vi "PDF_Interface_PDF Protokoll Linearisierung.vi"(2 "ResultPictures":T1, 3 "PDF Optionen":T2, 4 "Deckblatt_Name":string, 5 "start":bool, 6 "SpanComponentInfos-Cluster":T7, 7 "Save PDF File Path":path, 8 "error in (no error)":errorcluster caption="Fehler (Eingang, kein Fehler)", 9 "Context (Eingang)":refnum<class "Context.lvclass">, 10 "XY-Graph LIN":refnum<vi>, 11 "Polynom-Ordnung":T8) -> (0 "error out":errorcluster caption="Fehler (Ausgang)", 1 "Context (Ausgang)":refnum<class "Context.lvclass">)   [LabVIEW 2020, in "Linearisierung v2.lvlib" / "Protokoll.lvlib"]
uses:
  Protokoll.lvlib
  AktivArray.ctl
  AktivButton.ctl
  LIN Ausgabetabelle.ctl
  Polynomkoeffizientenanzeige.ctl
  Auswahl Polynom Ordnung.ctl
  <vilib>/Simplicity AI/SAI_PDF_API/Classes/Context/Context.lvclass
  SpanEinstellungen/SpanComponentInfos-Cluster.ctl
  SpanEinstellungen/ComponentInfos.ctl
  Visualisierungs Elemente/String - Ausgabefeld.ctl
  Visualisierungs Elemente/String - Eingabefeld.ctl
  SpanEinstellungen/PDF Optionen.ctl
  PDF_Interface/PDF Interface Helper/PDFResultPictures.ctl
  Sprachverwaltung/FGV Aktion Tabelle zerlegen.ctl
  Aktion Lin Daten aufarbeiten.ctl
  Seiten/FT-IR/FGV FT-IR Gasliste Aktionen.ctl
  Seiten/System Einstellungen V2/Aktion FGV SystemEinstellungenV2.ctl
  Gasteiler/Aktionen FGV Gasteiler Daten.ctl
  Seiten/System Einstellungen V2/Aktioen FGV System Konstanten.ctl
  Seiten/FT-IR/FGV FT-IR Aktionen.ctl
  PDF_Interface/PDF Protokoll Standard Kopf Optionen.ctl
  <vilib>/Simplicity AI/SAI_PDF_API/Classes/Context/Controls/SAI_PDF_PDF Details.ctl
  PDF_Interface/PDF Interface Helper/PDFGraph.ctl
  <vilib>/Simplicity AI/SAI_PDF_API/Classes/Context/Controls/SAI_PDF_Text Align.ctl
  PDF_Interface/PDF Interface Helper/PDFCommentPosition.ctl
  PDF_Interface/PDF Interface Helper/PDFPageBreak.ctl
  PDF_Interface/PDF Interface Helper/PDFContentType.ctl
  PDF_Interface/PDF Interface Helper/PDFTableContentType.ctl
  PDF_Interface/PDF Interface Helper/PDFResults.ctl
  PDF_Interface/PDF Interface Helper/PDFTablePictures.ctl
  PDF_Interface/PDF Interface Helper/PDFBemerkung.ctl
  <vilib>/Simplicity AI/SAI_PDF_API/Classes/Context/Controls/SAI_PDF_Font.ctl
  <vilib>/Simplicity AI/SAI_PDF_API/Classes/Context/Controls/SAI_PDF_Font Encoding.ctl
  PDF_Interface/PDF Interface Helper/PDFTtilePageContentType.ctl
  Gasteiler/HovaCAL_Interface/Kommunikation/Aktion FGV HovaCAL Interface Autolin.ctl
  GasteilerType.ctl
  Linearisierung v2.lvlib
  Allgemein/allgemeine Sub-VIs.lvlib
  Seiten/FT-IR/FT-IR.lvlib
  Seiten/System Einstellungen V2/System Einstellungen V2.lvlib
  Sprachverwaltung/Sprachverwaltung.lvlib
  PDF_Interface/PDF Interface.lvlib
  PDF_Interface/PDF Interface Helper/PDF Interface Helper.lvlib
  Gasteiler/Gasteiler.lvlib
  Gasteiler/HovaCAL_Interface/Kommunikation/Kommunikation.lvlib
  SpanEinstellungen/SpanEinstellungen.lvlib
panel:
  out "Gasflaschengenauigkeit":string caption="Genauigkeit:"
  out "Gasflaschennummer":string caption="Gasflasche:"
  out "Spanfaktor":string caption="Spanfaktor:"
  out "geforderte Genauigkeit":string caption="geforderte Genauigkeit:"
  out "Polynomkoeffizienten":T9 caption="Polynomkoeffizient:" {"O. 4" format="%#.10f"; "O. 3" format="%#.10f"; "O. 2" format="%#.10f"; "O.1" format="%#.10f"; "Offset" format="%#.10f"}
  out "Polynom-Ordnung":string caption="Polynom-Ordnung:"
  out "Ordnung festgelegt":string caption="Ordnung festgelegt:"
  out "erreichter max. Fehler (ppm)":string caption="erreichter max. Fehler (ppm):"
  out "erreichter max. Fehler (%)":string caption="erreichter max. Fehler (%):"
  out "geford. max. Fehler":string caption="geford. max. Fehler (% v. Sollw.):"
  out "LIN Ausgabetabelle":T10
  out "Aktiv":T11
  out "XY-Graph LIN":cluster{dbl[], dbl[]}[](graph) caption="XY-Graph"
  out "Datum:":string
  out "Konzentration:":string
  out "Komponente:":string
  out "Bearbeiter:":string
  out "Gasteiler:":string
  out "Messgerät:":string
  # "Linearity Check"
  # "Konstante"
  # "1.Ordnung"
  # "2.Ordnung"
  # "3.Ordnung"
  # "4.Ordnung"
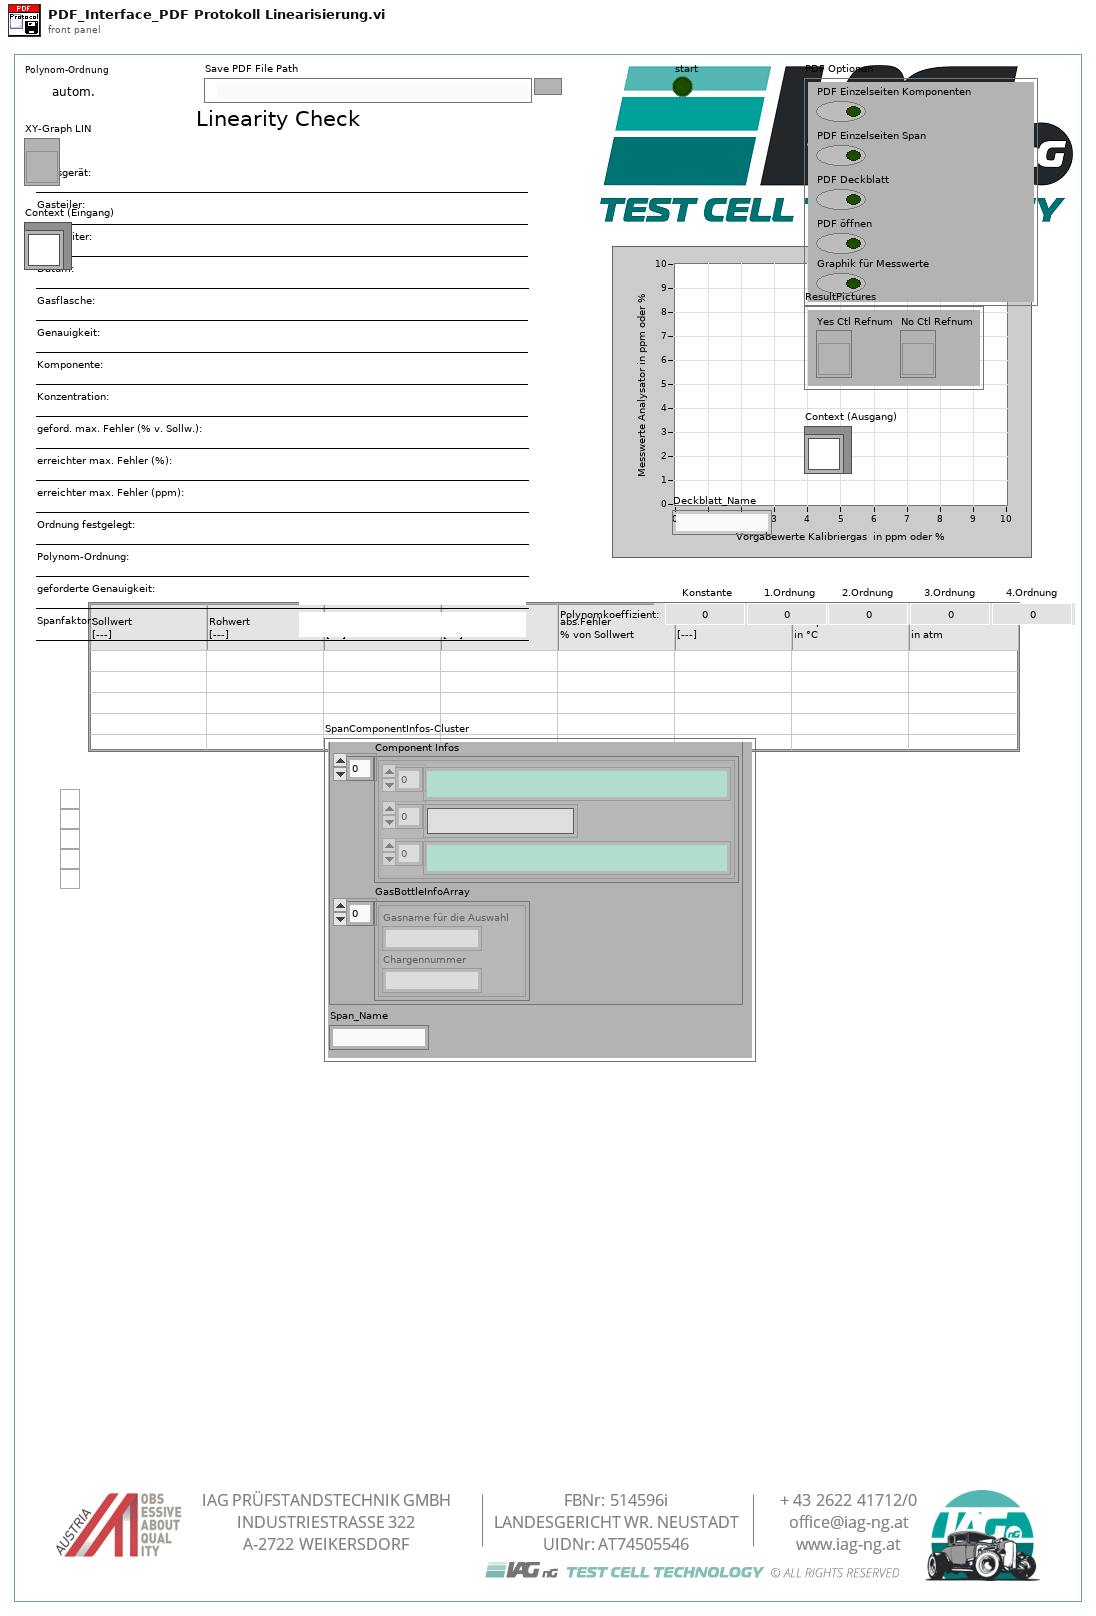
[diagram p1: front panel]
types:
  T1 = typedef "PDF Interface.lvlib/PDF Interface Helper.lvlib/PDFResultPictures.ctl" = cluster{"Yes Ctl Refnum":refnum<vi>, "No Ctl Refnum":refnum<vi>}
  T2 = typedef "Linearisierung v2.lvlib/SpanEinstellungen.lvlib/PDF Optionen.ctl" = cluster{"PDF Einzelseiten Komponenten":bool, "PDF Einzelseiten Span":bool, "PDF Deckblatt":bool, "PDF öffnen":bool, "Graphik für Messwerte":bool}
  T3 = typedef "Linearisierung v2.lvlib/SpanEinstellungen.lvlib/SpanComponentInfos-Cluster.ctl" = cluster{"SPAN Names":string[], "Component Infos":T4[], "GasBottleInfoArray":cluster{"Gasname für die Auswahl":string, "Chargennummer":string}[]}
  T4 = typedef "Linearisierung v2.lvlib/SpanEinstellungen.lvlib/ComponentInfos.ctl" = cluster{T5[], T6[], T5[]}
  T5 = typedef "String - Ausgabefeld.ctl" = string
  T6 = typedef "String - Eingabefeld.ctl" = string
  T7 = cluster{"SpanComponentInfos-Cluster":T3, "Span_Name":string}
  T8 = typedef "Linearisierung v2.lvlib/Auswahl Polynom Ordnung.ctl" = enum16{"autom.", "raw", "actual", "1", "2", "3", "4"}
  T9 = typedef "Linearisierung v2.lvlib/Polynomkoeffizientenanzeige.ctl" = cluster{"Offset":dbl, "O.1":dbl, "O. 2":dbl, "O. 3":dbl, "O. 4":dbl}
  T10 = typedef "Linearisierung v2.lvlib/LIN Ausgabetabelle.ctl" = string[][]
  T11 = typedef "Linearisierung v2.lvlib/AktivArray.ctl" = T12[]
  T12 = typedef "Linearisierung v2.lvlib/AktivButton.ctl" = bool
  T13 = typedef "Sprachverwaltung.lvlib/FGV Aktion Tabelle zerlegen.ctl" = enum16{"laden", "vereinzeln", "speichern"}
  T14 = typedef "PDF Interface.lvlib/PDF Protokoll Standard Kopf Optionen.ctl" = cluster{"Analysator":bool, "FT-IR Rezept":bool, "Gasteiler":bool, "Gas Komponente":bool, "Gas Flasche":bool, "LIN Protokoll":bool, "Operator":bool}
  T15 = typedef "FT-IR.lvlib/FGV FT-IR Aktionen.ctl" = enum16{"lesen", "NOG setzen", "NOS setzen", "Initialisieren", "speichern", "ALLES setzen", "FT-IR Spektrum loggen", "Komm Stoppen", "Spektrum LogKonfig"}
  T16 = typedef "System Einstellungen V2.lvlib/Aktioen FGV System Konstanten.ctl" = enum16{"lesen", "laden", "speichern", "Sprache"}
  T17 = typedef "Linearisierung v2.lvlib/Gasteiler.lvlib/Aktionen FGV Gasteiler Daten.ctl" = enum16{"lesen", "Gasteiler Daten", "Seriellen Param.", "MB-Endwert", "laden", "speichern", "Anforderung", "TCP", "Aufzeichnung Start"}
  T18 = typedef "System Einstellungen V2.lvlib/Aktion FGV SystemEinstellungenV2.ctl" = enum16{"lesen", "Analysatoren schreiben", "Analysator ändern", "Analysatoren löschen", "laden", "speichern", "Untertitel", "Analysatoren", "Neue Analysatoren", "Gasteiler schreiben", "Gasteiler ändern", "Gasteiler löschen", "Gasteiler", "Gasteiler exportieren", "Gasteiler importieren"}
  T19 = typedef "FT-IR.lvlib/FGV FT-IR Gasliste Aktionen.ctl" = enum16{"lesen", "Gasliste FT-IR", "Gasliste ausgelesen", "laden", "speichern", "löschen"}
  T20 = typedef "Linearisierung v2.lvlib/Aktion Lin Daten aufarbeiten.ctl" = enum16{"lesen", "Protkolldaten", "speichern", "laden", "EPA auswerten", "Tabelle schreiben", "Lin auswerten", "Tab init", "Stufentabelle", "EPA aktiviert", "Nachbehandlung laden", "Tabelle löschen", "Istwerte löschen", "Zeile löschen", "Zeile einfügen", "LIN aktiviert", "LIN/EPA aktiv laden", "EGAK Tab", "LIN übernehmen", "Tab init ohne Stufen"}
  T21 = typedef "PDF Interface.lvlib/PDF Interface Helper.lvlib/PDFPageBreak.ctl" = enum16{"none", "before", "after", "after comment"}
  T22 = typedef "PDF Interface.lvlib/PDF Interface Helper.lvlib/PDFCommentPosition.ctl" = enum16{"before", "after"}
  T23 = typedef "Linearisierung v2.lvlib/Gasteiler.lvlib/HovaCAL_Interface.lvlib/Kommunikation.lvlib/Aktion FGV HovaCAL Interface Autolin.ctl" = enum16{"lesen", "schreiben", "MFC Komponente fix setzen", "init"}
  T24 = typedef "SAI_PDF_Toolkit.lvlib/Context.lvclass/SAI_PDF_Font.ctl" = cluster{"Font":string, "Size":i32, "Colour":u32, "Bold":bool, "Italic":bool, "Underline":bool, "Strikethrough":bool, "Font Encoding":T25}
  T25 = typedef "SAI_PDF_Toolkit.lvlib/Context.lvclass/SAI_PDF_Font Encoding.ctl" = enum16{"Cp1252, WinANSI", "IdentityH", "IdentityV", "Cp1250", "Cp1257", "MacRoman"}
  T26 = typedef "PDF Interface.lvlib/PDF Interface Helper.lvlib/PDFBemerkung.ctl" = cluster{"Bemerkung Text":string, "Align (Left)":T27, "Add Line Feeds (F:No)":bool, "Font":T24}
  T27 = typedef "SAI_PDF_Toolkit.lvlib/Context.lvclass/SAI_PDF_Text Align.ctl" = i32
  T28 = typedef "PDF Interface.lvlib/PDF Interface Helper.lvlib/PDFTableContentType.ctl" = cluster{"TableHeader":string[], "Table":string[][], "Relative Column Widths (%)":sgl[], "Results":T29, "PositionBemerkung":T22, "PageBreak":T21, "TablePictures":T30, "Horizontal Align":i32}
  T29 = typedef "PDF Interface.lvlib/PDF Interface Helper.lvlib/PDFResults.ctl" = cluster{"Results":cluster{"Result Text":string, "Result":bool}[], "ResultPictures":T1, "use Pictures":bool, "Image Scale (%)":sgl, "Autoscale? (T)":bool, "Horizontal Align":i32, "Position":i32}
  T30 = typedef "PDF Interface.lvlib/PDF Interface Helper.lvlib/PDFTablePictures.ctl" = cluster{"Ctl Refnum In":refnum<vi>[], "RowOrColumn":enum16{"Row", "Column"}, "IndexToInsert":u16, "Image Scale (%)":sgl[], "Autoscale? (T)":bool[], "Horizontal Align":i32}
  T31 = typedef "PDF Interface.lvlib/PDF Interface Helper.lvlib/PDFTtilePageContentType.ctl" = cluster{"Titel":string, "Header Tables":string[][][], "Bemerkungen":T26[]}
  T32 = typedef "PDF Interface.lvlib/PDF Interface Helper.lvlib/PDFContentType.ctl" = cluster{"Titel":string, "Header Table":string[][], "Table Array":T28[], "Bemerkungen":T26[]}
  T33 = typedef "PDF Interface.lvlib/PDF Interface Helper.lvlib/PDFGraph.ctl" = cluster{"GraphCtl Refnum":refnum<vi>, "Wrap Text (F:No)":bool, "Hide Grid (F:No)":bool, "Scale (100%)":sgl, "Align (Left)":T27, "PositionBemerkung":T22, "PageBreak":T21}
  T34 = typedef "SAI_PDF_Toolkit.lvlib/Context.lvclass/SAI_PDF_PDF Details.ctl" = cluster{"Title":string, "Subject":string, "Keywords":string, "Author":string, "Creator":string}
  T35 = cluster{"Header Footer Text Cluster":cluster{"Header Text":string, "Footer Text":string, "Time":string, "Page Number":string}, "PDF Details":T34}
  T36 = typedef "System Einstellungen V2.lvlib/Gasteiler.ctl" = cluster{"Gasteiler Name":string, "Gasteiler Type":string, "Gasteiler Seriennummer":string, "Gasteiler Letzte Wartung":timestamp}
  T37 = cluster{"GasteilerDefinitionsListe":T36[], "GasteilerDefinitionTextliste":string[][], "Gasteiler Strings And Values":cluster{"String":string, "Wert":string}[]}
  T38 = typedef "Linearisierung v2.lvlib/Gasteiler.lvlib/Gasteiler Daten.ctl" = cluster{"Gasteiler":T6, "Gasteiler Stufen":T39, "Gasteiler Type":T40, "Konfig Gasteiler":T41, "Gasteiler Span Eingänge":u16}
  T39 = typedef "Linearisierung v2.lvlib/Gasteiler.lvlib/Gasteiler Stufen.ctl" = u16
  T40 = typedef "Linearisierung v2.lvlib/GasteilerType.ctl" = u16
  T41 = typedef "System Einstellungen V2.lvlib/Gasteiler Auswahl.ctl" = u16
  T42 = typedef "Auswahlfeld.ctl" = u16
  T43 = cluster{"Modell":string, "ProjektNummer":string, "Software Version":string, "Seriennummer":string}
  T44 = typedef "Linearisierung v2.lvlib/Eingabetabelle.ctl" = string[][]
  T45 = typedef "Linearisierung v2.lvlib/Lin-Polynom Daten.ctl" = cluster{"Messgerät":string, "Kalibrator (Gasteiler)":string, "Bearbeiter/in":string, "Komponente":string, "Zeitstempel":timestamp, "F_max gefordert (%)":sgl, "F_max in %":sgl, "F_max in ppm":sgl, "Vorschlag Ordnung":i32, "Polynom OK":bool, "Polynomkoeff.":dbl[], "Prüfgas Konzentration":dbl, "Pfad EPA":string, "Pfad_LIN":string, "Gasnummer:":u8, "Komponentenauswahl":T46, "Verdünnungsgas":T47, "Zeitdauer Stufe":T48, "Anzahl Stufen":T48, "F_max in % EPA":sgl, "F_max in ppm EPA":sgl, "F_max in % LIN":sgl, "F_max in ppm LIN":sgl, "Punkte umkehren":bool, "EPA Optionsfeld":T49, "Autolin Hovacal":T50, "Spanfactors":sgl[], "Kalibrierauswahl":T51, "Conditions:":T52, "Gasflaschen Nr.:":string, "Bottle Accuracy":dbl, "Konfig Gasflasche":T53, "Gasflasche":T54, "HovaCAL Flow AutoLin":T55, "MFC Output":T56, "Gas Ablaufdatum":timestamp, "Lin Modus":T57, "zusätzliche Zeitdauer Erster Punkt":sgl, "Offsets":sgl[]}
  T46 = typedef "Linearisierung v2.lvlib/KomponentenArray.ctl" = cluster{"Komponente:":T42, "Konzentration":dbl}[]
  T47 = typedef "Linearisierung v2.lvlib/Gasteiler.lvlib/Prüfgas in.ctl" = u16
  T48 = typedef "Zahlen-Eingabefeld.ctl" = sgl
  T49 = typedef "Linearisierung v2.lvlib/EPA Optionsfeld.ctl" = enum32{"Istwert", "Rohwert", "Linearisierter Wert"}
  T50 = typedef "Linearisierung v2.lvlib/Gasteiler.lvlib/HovaCal.lvlib/AutoLin Hovacal.ctl" = enum32{"Keine Auswahl", "Optionsauswahl 1", "Optionsauswahl 2"}
  T51 = typedef "Linearisierung v2.lvlib/Kalibrieroption.ctl" = u16
  T52 = typedef "Linearisierung v2.lvlib/Linearity verification 1065-307.lvlib/Condition.ctl" = u16
  T53 = typedef "System Einstellungen V2.lvlib/Konfig Gasflasche.ctl" = bool
  T54 = typedef "System Einstellungen V2.lvlib/Gasflasche Auswahl.ctl" = u16
  T55 = typedef "Linearisierung v2.lvlib/Gasteiler.lvlib/HovaCAL_Interface.lvlib/Controls.lvlib/Flow Einstellung.ctl" = cluster{"HovaCAL Flow Input Cluster":dbl}
  T56 = typedef "Linearisierung v2.lvlib/Gasteiler.lvlib/HovaCAL_Interface.lvlib/Controls.lvlib/Pump state.ctl" = cluster{"Run":bool}
  T57 = typedef "CalGas Aufschaltung.lvlib/Lin Modus.ctl" = u16
  T58 = cluster{"Polynomkoeff.[0]":dbl, "Polynomkoeff.[1]":dbl, "Polynomkoeff.[2]":dbl, "Polynomkoeff.[3]":dbl, "Polynomkoeff.[4]":dbl}
  T59 = cluster{"Header Size":i32, "Column Ratio left":sgl[]}
  T60 = cluster{"Dieses VI":refnum<vi>, "Cluster (Eingang)":refnum<vi>, "Graphik (Eingang)":refnum<vi>, "Clear (Eingang)":refnum<vi>}
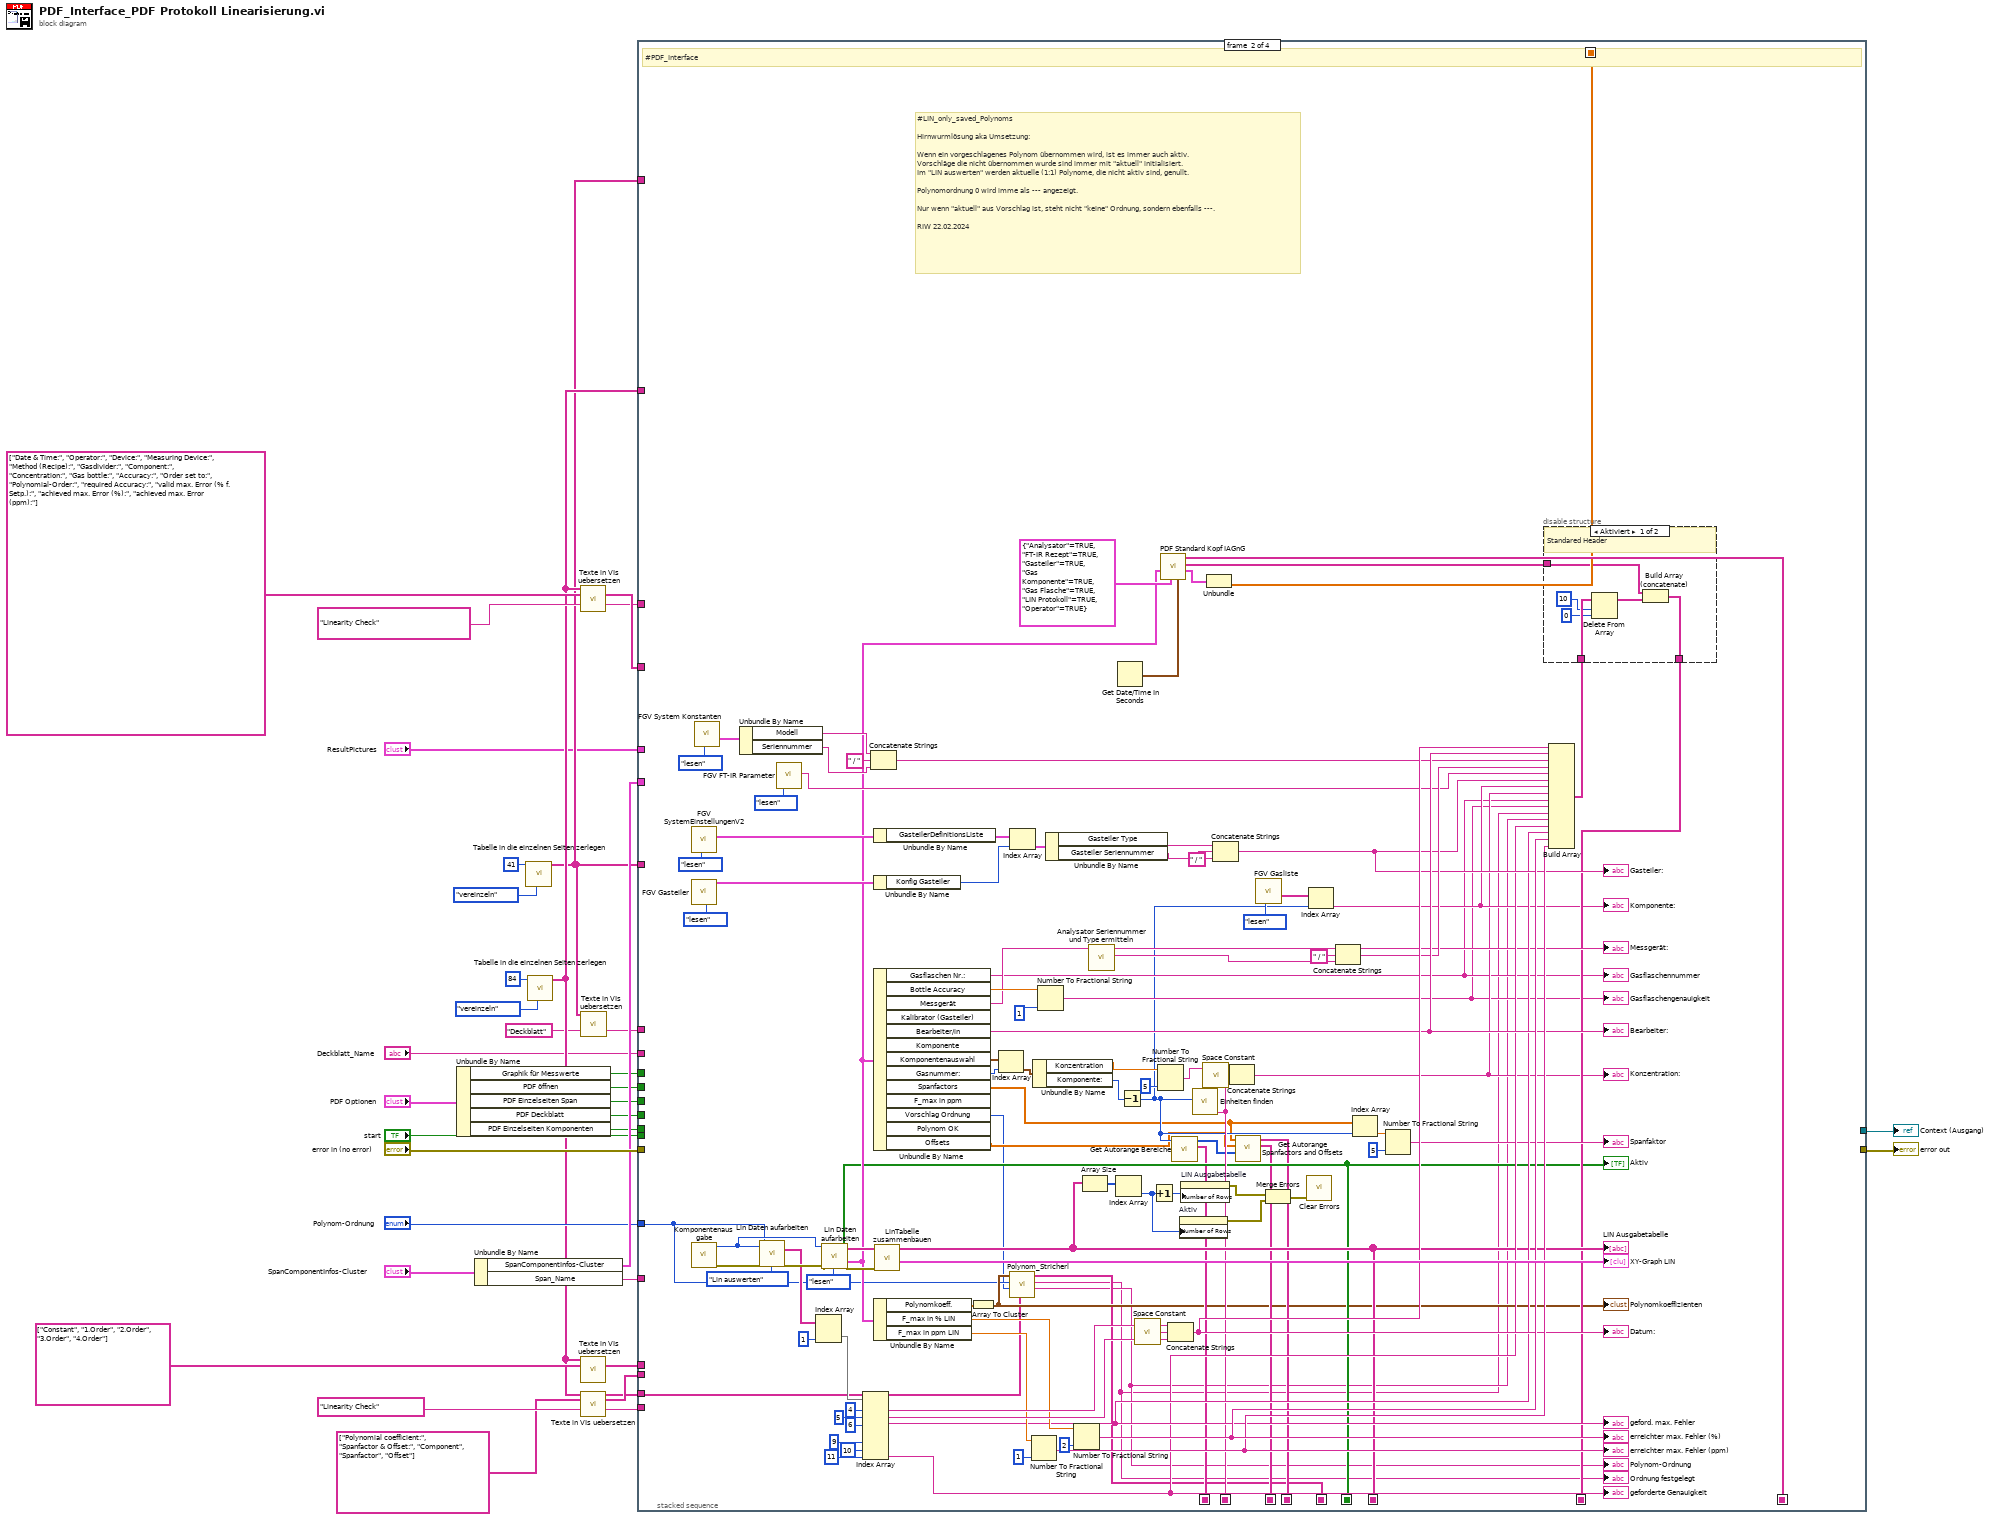
[diagram p0: block diagram]
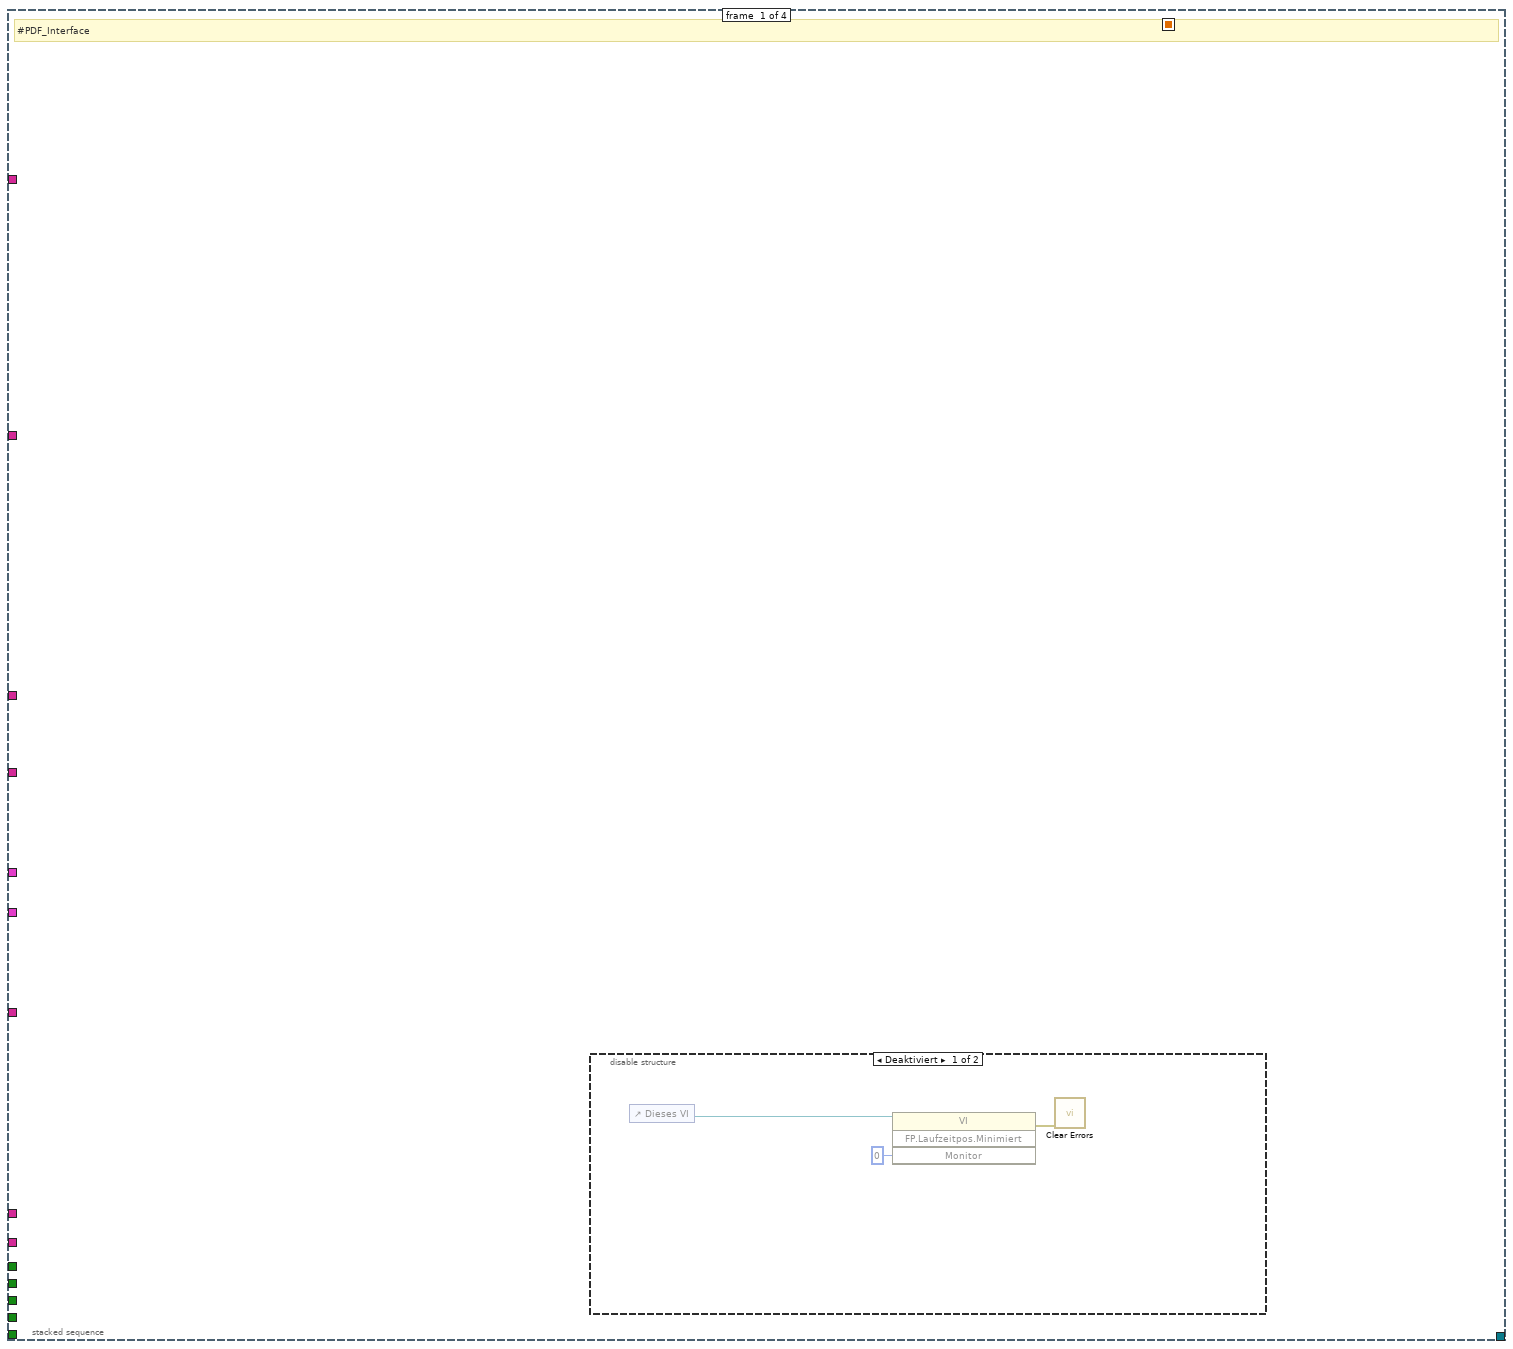
[diagram p2: hidden frame]
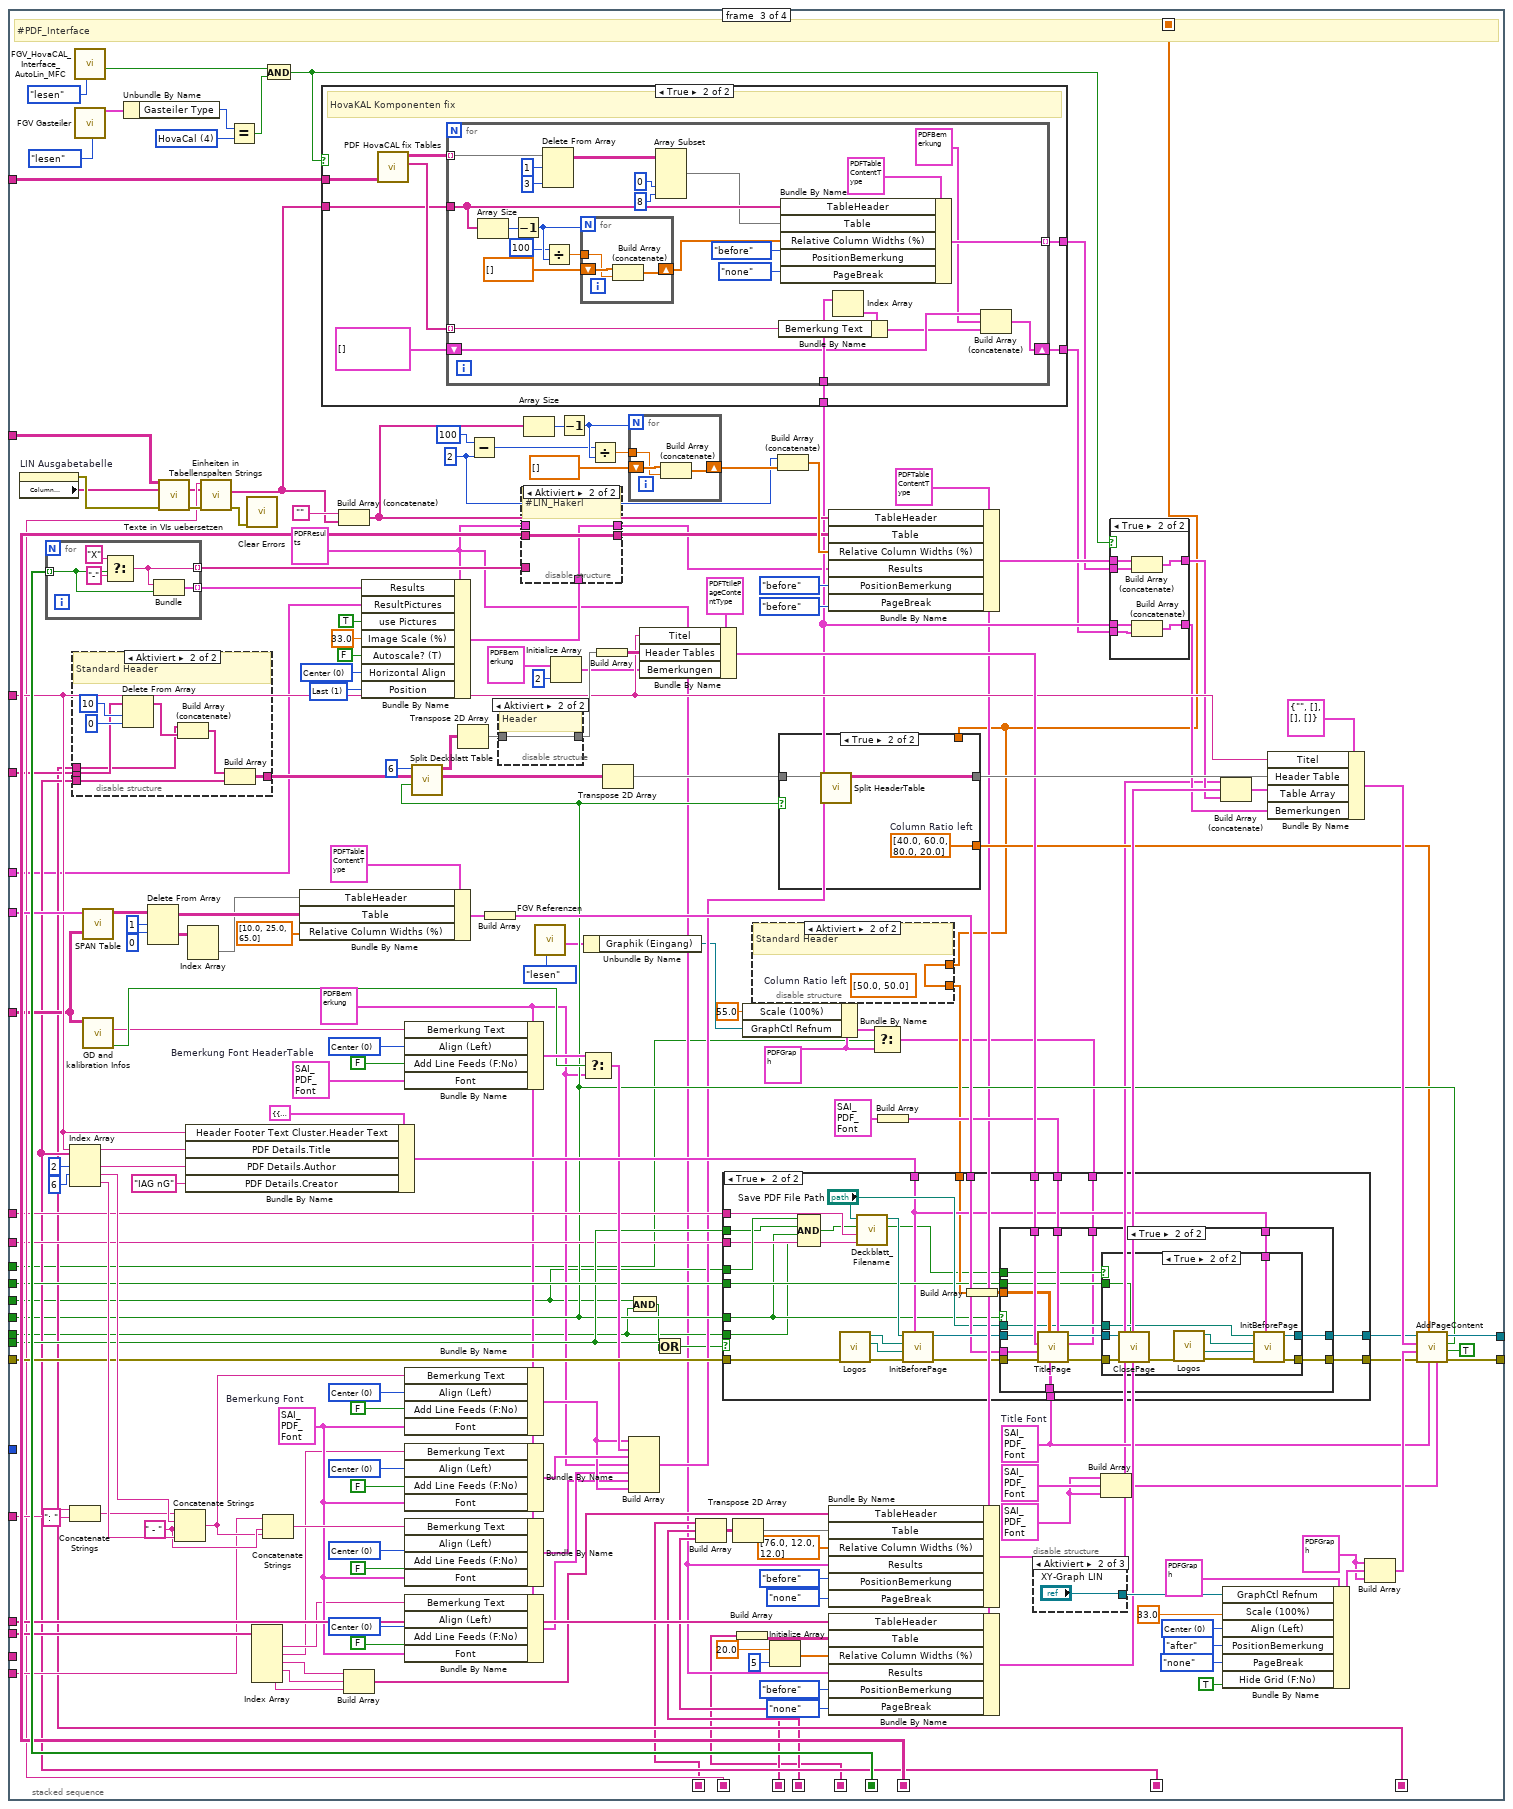
[diagram p5: hidden frame]
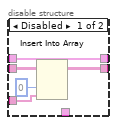
[diagram p6: hidden frame]
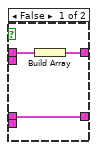
[diagram p8: hidden frame]
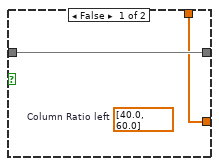
[diagram p9: hidden frame]
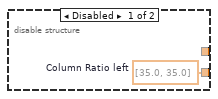
[diagram p10: hidden frame]
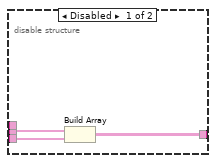
[diagram p11: hidden frame]
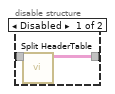
[diagram p12: hidden frame]
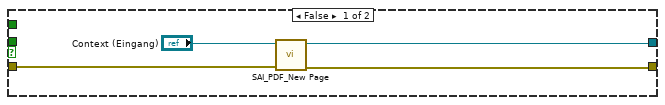
[diagram p13: hidden frame]
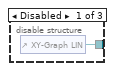
[diagram p16: hidden frame]
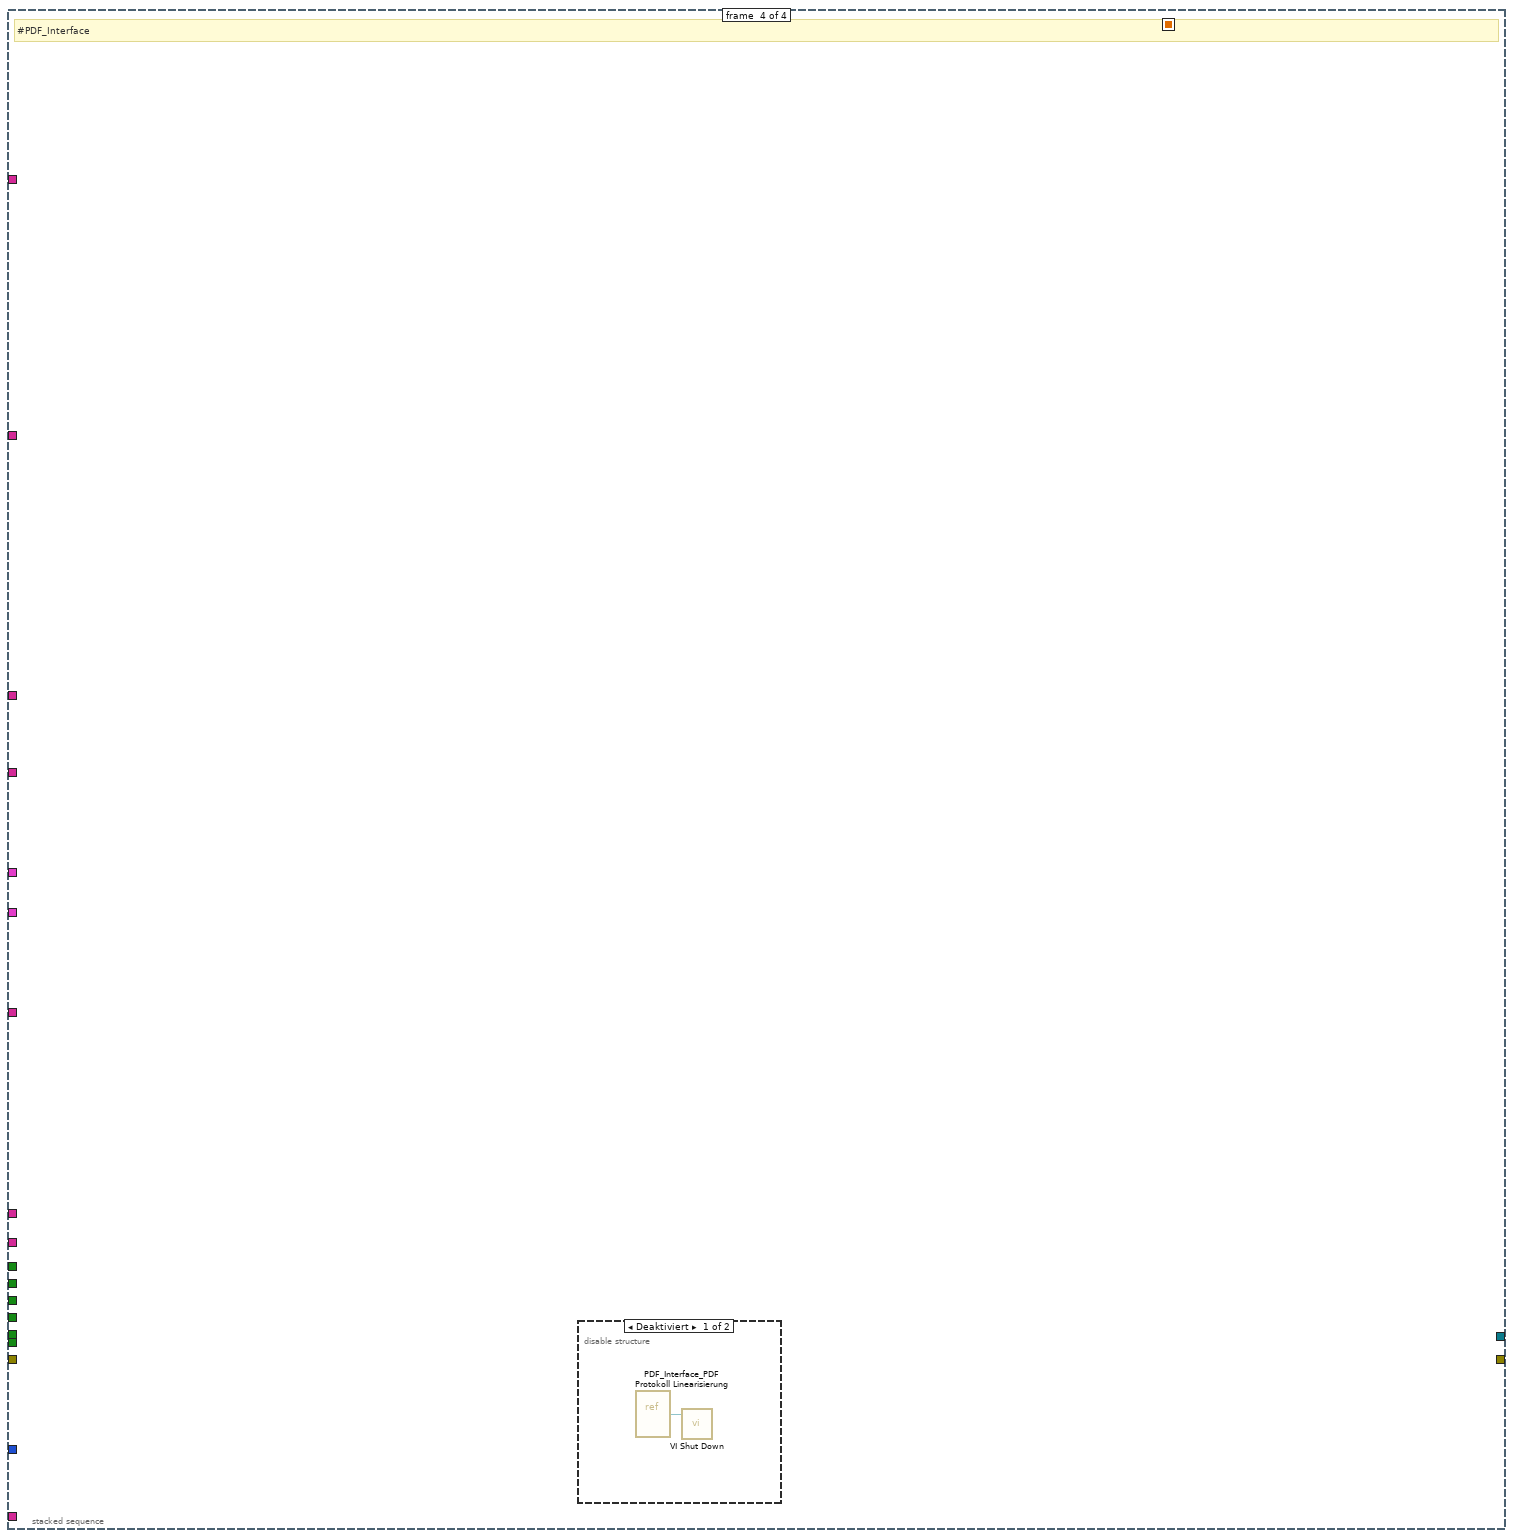
[diagram p18: hidden frame]
diagram:
  n1 = Unbundle By Name("PDF Optionen") -> ("Graphik für Messwerte"=w1:bool, "PDF öffnen"=w11:bool, "PDF Einzelseiten Span"=w12:bool, "PDF Deckblatt"=w13:bool, "PDF Einzelseiten Komponenten"=w3:bool)
  n2 = Unbundle By Name("SpanComponentInfos-Cluster") -> ("SpanComponentInfos-Cluster"=w30:T3, "Span_Name"=w31:string)
  n3 = call "Tabelle in die einzelnen Seiten zerlegen.vi"("Aktion"=FGV_Aktion_Tabelle_zerlegen."vereinzeln", "Index (Seite)"=41) -> ("Sprachliste"=w7:string[][])  [unwired: 7 in, 2 out]
  n4 = call "Tabelle in die einzelnen Seiten zerlegen.vi"("Aktion"=FGV_Aktion_Tabelle_zerlegen."vereinzeln", "Index (Seite)"=84) -> ("Sprachliste"=w15:string[][])  [unwired: 7 in, 2 out]
  n5 = call "Texte in VIs uebersetzen.vi"("Sprachliste"=w15, "String-Array zum Übersetzen"=string[] ["Date & Time:", "Operator:", "Device:", "Measuring Device:", "Method (Recipe):", "Gasdivider:", "Component:", "Concentration:", "Gas bottle:", "Accuracy:", "Order set to:", "Polynomial-Order:", "required Accuracy:", "valid max. Error (% f. Setp.):", "achieved max. Error (%):", "achieved max. Error (ppm):"], "String zum Übersetzen"="Linearity Check") -> ("String-Array zum Übersetzen"=w27:string[], "String zum Übersetzen"=w26:string)  [unwired: 8 in, 3 out]
  n6 = call "Texte in VIs uebersetzen.vi"("Sprachliste"=w15, "String-Array zum Übersetzen"=string[] ["Constant", "1.Order", "2.Order", "3.Order", "4.Order"] ("String")) -> ("String-Array zum Übersetzen"=w20:string[])  [unwired: 9 in, 4 out]
  n7 = call "Texte in VIs uebersetzen.vi"("Sprachliste"=w15, "String-Array zum Übersetzen"=string[] ["Polynomial coefficient:", "Spanfactor & Offset:", "Component", "Spanfactor", "Offset"] ("String"), "String zum Übersetzen"="Linearity Check" ("String")) -> ("Sprachliste out"=w4:string[][], "String-Array zum Übersetzen"=w5:string[], "String zum Übersetzen"=w16:string)  [unwired: 8 in, 2 out]
  n8 = call "Texte in VIs uebersetzen.vi"("Sprachliste"=w7, "String zum Übersetzen"="Deckblatt") -> ("String zum Übersetzen"=w9:string)  [unwired: 9 in, 4 out]
  n9 = stacked-sequence {
    seq-local: [_ w63 _ _] -> [_ _ w229 _]
    seq-local: [_ w72 _ _] -> [_ _ w335 _]
    seq-local: [_ w56 _ _] -> [_ _ w337 _]
    seq-local: [_ w44 _ _] -> [_ _ w160 _]
    seq-local: [_ w71 _ _] -> [_ _ w237 _]
    seq-local: [_ w62 _ _] -> [_ _ w226 _]
    seq-local: [_ w51 _ _] -> [_ _ w181 _]
    seq-local: [_ w50 _ _] -> [_ _ w180 _]
    seq-local: [_ w49 _ _] -> [_ _ w178 _]
    seq-local: [_ w46 _ _] -> [_ _ w176 _]
    tunnel: "error in (no error)" -> [_ _ w288 _]
    tunnel: [_ _ w328 _] -> w34
    tunnel: [_ _ w287 _] -> w33
    tunnel: w31 -> [_ _ w266 _]
    tunnel: w30 -> [_ _ w265 _]
    tunnel: "Polynom-Ordnung" -> [_ w43 _ _]
    tunnel: w27 -> [_ _ w228 _]
    tunnel: w26 -> [_ _ w251 _]
    tunnel: w7 -> [_ _ w232 _]
    tunnel: w20 -> [_ _ w250 _]
    tunnel: w5 -> [_ _ w249 _]
    tunnel: w16 -> [_ _ w248 _]
    tunnel: w13 -> [_ _ w224 _]
    tunnel: "start" -> [_ _ w235 _]
    tunnel: w15 -> [_ _ w206 _]
    tunnel: w12 -> [_ _ w174 _]
    tunnel: w11 -> [_ _ w236 _]
    tunnel: w9 -> [_ _ w234 _]
    tunnel: "Deckblatt_Name" -> [_ _ w233 _]
    tunnel: w7 -> [_ _ w205 _]
    tunnel: w4 -> [_ w41 _ _]
    tunnel: w3 -> [_ _ w172 _]
    tunnel: "ResultPictures" -> [_ _ w164 _]
    tunnel: w1 -> [_ _ w156 _]
    frame #0 {
      # "#PDF_Interface"
      n10 = disable-structure shown="Deaktiviert" {
        frame Disabled {
          n11 = control-ref of="Dieses VI"() -> (w38:refnum<vi>)
          n12 = invoke class="VI" method="FP.Laufzeitpos.Minimiert"(reference=w38, "Monitor"=i16 0) -> (error out=w36:errorcluster)  [unwired: 2 in, 3 out]
          n13 = call <vilib>:"Clear Errors.vi"("error in (no error)"=w36) -> ()  [unwired: 5 in, 2 out]
        }
        frame Enabled {
        }
      }
    }
    frame #1 {
      # "#LIN_only_saved_Polynoms\n\nHirnwurmlösung aka Umsetzung:\n\nWenn ein vorgeschlagenes Polynom übernommen wird, ist es immer auch aktiv.\nVorschläge die nicht übernommen wurde sind immer mit \"aktuell\" initialisiert.\nIm \"LIN auswerten\" werden aktuelle (1:1) Polynome, die nicht aktiv sind, genullt.\n\nPolynomordnung 0 wird imme als --- angezeigt.\n\nNur wenn \"aktuell\" aus Vorschlag ist, steht nicht \"keine\" Ordnung, sondern ebenfalls ---.\n\nRIW 22.02.2024"
      # "#PDF_Interface"
      n14 = call "FGV SystemEinstellungenV2.vi"("Aktion"=Aktion_FGV_SystemEinstellungenV2."lesen") -> ("Gasteiler"=w99:T37)  [unwired: 5 in, 5 out]
      n15 = call "FGV Gasteiler.vi"("Aktionen"=Aktionen_FGV_Gasteiler_Daten."lesen") -> ("Gasteiler Daten"=w97:T38)  [unwired: 11 in, 7 out]
      n16 = call "Komponentenausgabe.vi"() -> ("error out"=w137:errorcluster, "Gaskomponente"=w70:T42)  [unwired: 8 in, 2 out]
      n17 = call "FGV System Konstanten.vi"("Aktionen"=Aktioen_FGV_System_Konstanten."lesen") -> ("Cluster out"=w87:T43)  [unwired: 6 in, 4 out]
      n18 = Unbundle By Name(w87) -> ("Modell"=w84:string, "Seriennummer"=w83:string)
      n19 = call "Lin Daten aufarbeiten.vi"("Index (Seite)"=w70, "error in (no error)"=w137, "Polynom-Ordnung"=w43, "Aktionen"=Aktion_Lin_Daten_aufarbeiten."Lin auswerten") -> ("Ergebnis Lin"=w133:string[][], "error out"=w142:errorcluster)  [unwired: 13 in, 9 out]
      n20 = call "FGV FT-IR Parameter.vi"("Aktion"=FGV_FT-IR_Aktionen."lesen") -> ("Current Recipe"=w77:string)  [unwired: 11 in, 7 out]
      n21 = Index Array(array=w133, index (col)=1 ("Deaktivierter Index (Spalte)")) -> (element=w131:string[])  [unwired: 1 in]
      n22 = call "Lin Daten aufarbeiten.vi"("Index (Seite)"=w70, "error in (no error)"=w142, "Aktionen"=Aktion_Lin_Daten_aufarbeiten."lesen") -> ("Aktiv LIN"=w56:bool[], "Eingabetabelle"=w135:T44, "Lin-Polynom"=w66:T45, "error out"=w134:errorcluster)  [unwired: 14 in, 7 out]
      "Aktiv" <- w56
      n23 = Index Array(array=w131, index #1=4 ("Index"), index #2=5 ("Index"), index #3=6 ("Index"), index #6=9 ("Index"), index #7=10 ("Index"), index #8=11 ("Index")) -> (element #1=w128:string, element #2=w126:string, element #3=w75:string, element #8=w74:string)  [unwired: 2 in, 4 out]
      "geford. max. Fehler" <- w75
      "geforderte Genauigkeit" <- w74
      n24 = Concatenate Strings(w84, " / " ("String"), w83) -> (w79:string)
      n25 = Unbundle By Name(w99) -> ("GasteilerDefinitionsListe"=w98:T36[])
      n26 = Unbundle By Name(w97) -> ("Konfig Gasteiler"=w96:T41)
      n27 = Unbundle By Name(w66) -> ("Gasflaschen Nr.:"=w59:string, "Bottle Accuracy"=w105:dbl, "Messgerät"=w104:string, "Bearbeiter/in"=w80:string, "Komponentenauswahl"=w141:T46, "Gasnummer:"=w140:u8, "Spanfactors"=w53:sgl[], "Vorschlag Ordnung"=w42:i32, "Offsets"=w52:sgl[])  [unwired: 4 out]
      "Bearbeiter:" <- w80
      "Gasflaschennummer" <- w59
      n28 = Unbundle By Name(w66) -> ("Polynomkoeff."=w57:dbl[], "F_max in % LIN"=w115:sgl, "F_max in ppm LIN"=w114:sgl)
      n29 = call "LinTabelle zusammenbauen.vi"("error in (no error)"=w134, "Eingabetabelle"=w135) -> ("XY-Graph"=→"XY-Graph LIN":cluster{dbl[], dbl[]}[], "LIN Ausgabetabelle"=w72:string[][])  [unwired: 6 in, 2 out]
      "LIN Ausgabetabelle" <- w72
      n30 = Array To Cluster(array=w57) -> (cluster=w45:T58)
      "Polynomkoeffizienten" <- w45
      n31 = Index Array(array=w141, index=w140) -> (element=w139:cluster{"Komponente:":T42, "Konzentration":dbl})
      n32 = call "Polynom_Stricherl.vi"("Sprachliste"=w41, "Vorschlag Ordnung"=w42, "Polynom-Ordnung"=w43, "Polynomkoeff."=w45) -> ("Vorschlag Ordnung String"=w40:string, "Ordnung festgelegt String"=w39:string, "Polynom String Array"=w44:string[])  [unwired: 4 in, 1 out]
      "Polynom-Ordnung" <- w40
      "Ordnung festgelegt" <- w39
      n33 = Index Array(array=w98, index=w96) -> (element=w95:T36)
      n34 = Number To Fractional String(number=w114, precision (6)=i16 1 ("Genauigkeit (6)")) -> (F-format string=w101:string)  [unwired: 2 in]
      "erreichter max. Fehler (ppm)" <- w101
      n35 = Unbundle By Name(w139) -> ("Konzentration"=w138:dbl, "Komponente:"=w111:T42)
      n36 = Number To Fractional String(number=w105, precision (6)=i16 1 ("Genauigkeit (6)")) -> (F-format string=w58:string)  [unwired: 2 in]
      "Gasflaschengenauigkeit" <- w58
      n37 = Unbundle By Name(w95) -> ("Gasteiler Type"=w93:string, "Gasteiler Seriennummer"=w92:string)
      n38 = Number To Fractional String(number=w115, precision (6)=i16 2 ("Genauigkeit (6)")) -> (F-format string=w102:string)  [unwired: 2 in]
      "erreichter max. Fehler (%)" <- w102
      n39 = Array Size(array=w72) -> (size(s)=w121:i32[])
      n40 = call "Analysator Seriennummer und Type ermitteln.vi"("Analysator"=w104) -> ("Type"=w68:string, "Name für Protokoll"=w69:string)  [unwired: 8 in, 1 out]
      "Messgerät:" <- w69
      n41 = Index Array(array=w121) -> (element=w119:i32)  [unwired: 1 in]
      n42 = Get Date/Time In Seconds() -> (seconds since 1Jan1904=w48:timestamp)
      n43 = Decrement(x=w111) -> (x-1=w55:T42)
      n44 = call <vilib>:"Space Constant.vi"() -> ("String"=w127:string)
      n45 = Increment(x=w119) -> (x+1=w120:i32)
      n46 = Number To Fractional String(number=w138, precision (6)=i16 5 ("Genauigkeit (6)")) -> (F-format string=w89:string)  [unwired: 2 in]
      n47 = call "PDF Standard Kopf IAGnG.vi"("Zeitstempel"=w48, "Oprtionen Cluster"=T14 {"Analysator"=TRUE, "FT-IR Rezept"=TRUE, "Gasteiler"=TRUE, "Gas Komponente"=TRUE, "Gas Flasche"=TRUE, "LIN Protokoll"=TRUE, "Operator"=TRUE}, "LIN Pototokoll-Cluster (opotional)"=w66) -> ("Size Cluster"=w47:T59, "Header Values"=w65:T5[], "Header Labels"=w62:string[])  [unwired: 5 in, 1 out]
      n48 = Concatenate Strings(w128, w127, w126) -> (w81:string)
      "Datum:" <- w81
      n49 = call "Get Autorange Bereiche.vi"("Gaskomponente"=w55) -> (2:"Autorange Bereiche"=w49:T5[], 3:"Autorange Bereiche"=w54:T42[])  [unwired: 8 in, 1 out]
      n50 = property on="Aktiv" class="Arr"("Number of Rows"=w119) -> (error out=w117:errorcluster)  [unwired: 2 in, 1 out]
      n51 = property on="LIN Ausgabetabelle" class="Tbl (strikt)"("Number of Rows"=w120) -> (error out=w118:errorcluster)  [unwired: 2 in, 1 out]
      n52 = call "Einheiten finden.vi"("Komponente"=w55) -> ("Einheit in String"=w71:string)  [unwired: 6 in, 4 out]
      n53 = call <vilib>:"Space Constant.vi"() -> ("String"=w88:string)
      n54 = Unbundle(w47) -> ("Column Ratio left"=w46:sgl[])  [unwired: 1 out]
      n55 = Concatenate Strings(w93, " / " ("String"), w92) -> (w76:string)
      "Gasteiler:" <- w76
      n56 = Concatenate Strings(w89, w88, w71) -> (w60:string)
      "Konzentration:" <- w60
      n57 = call "Get Autorange Spanfactors and Offsets.vi"("Autorange Bereiche"=w54, "Offset"=w52, "Span"=w53) -> ("Autorange Offsets"=w50:string[], "Autorange Spanfactors"=w51:string[])  [unwired: 4 in, 3 out]
      n58 = call "FGV Gasliste.vi"("Aktionen"=FGV_FT-IR_Gasliste_Aktionen."lesen") -> ("Aktuelle Gasliste gesamt"=w103:T5[])  [unwired: 8 in, 2 out]
      n59 = Merge Errors(w118, w117) -> (w116:errorcluster)
      n60 = call <vilib>:"Clear Errors.vi"("error in (no error)"=w116) -> ()  [unwired: 5 in, 2 out]
      n61 = Index Array(array=w103, index=w55) -> (element=w61:T5)
      "Komponente:" <- w61
      n62 = Concatenate Strings(w69, " / " ("String"), w68) -> (w78:string)
      n63 = Index Array(array=w53, index=w55) -> (element=w108:sgl)
      n64 = Number To Fractional String(number=w108, precision (6)=i16 5 ("Genauigkeit (6)")) -> (F-format string=→"Spanfaktor":string)  [unwired: 2 in]
      n65 = Build Array(w81, w80, w79, w78, w77, w76, w61, w60, w59, w58, w39, w40, w74, w75, w102, w101) -> (w64:T5[])
      n66 = disable-structure shown="Aktiviert" {
        disable-tunnel: w64 -> [w150 w151]
        disable-tunnel: w65 -> [w145 _]
        disable-tunnel: [w146 w151] -> w63
        frame Enabled {
          # "Standared Header"
          n67 = Delete From Array(array=w150, length=10 ("Länge"), index=0 ("Index")) -> (array with subset deleted=w149:T5[])  [unwired: 1 out]
          n68 = Build Array (concatenate)(w145, w149) -> (w146:T5[])
        }
        frame Disabled {
        }
      }
    }
    frame #2 {
      w158 = T33 {"GraphCtl Refnum"=refnum, "Wrap Text (F:No)"=FALSE, "Hide Grid (F:No)"=FALSE, "Scale (100%)"=60.0, "Align (Left)"=0, "PositionBemerkung"=enum."before", "PageBreak"=enum."none"} ("Graph")
      w161 = 1 items=["First", "Last"] ("Position")
      w168 = T27 0 items=["Center", "Justified", "Justified All", "Left", "Right"] ("Align (Left)")
      w201 = T27 0 items=["Center", "Justified", "Justified All", "Left", "Right"] ("Align (Left)")
      w217 = T40 4 items=["LNI", "Analog-Display", "AVL GDU", "Horiba GDC", "HovaCal", "Horiba SGD 710C"] ("y")
      w189 = T24 {"Font"="Arial", "Size"=10, "Colour"=0, "Bold"=FALSE, "Italic"=FALSE, "Underline"=FALSE, "Strikethrough"=FALSE, "Font Encoding"=enum."Cp1252, WinANSI"} ("TableFont")
      w199 = T24 {"Font"="Arial", "Size"=12, "Colour"=0, "Bold"=TRUE, "Italic"=TRUE, "Underline"=FALSE, "Strikethrough"=FALSE, "Font Encoding"=enum."Cp1252, WinANSI"}  # Bemerkung Font
      w240 = T24 {"Font"="Arial", "Size"=12, "Colour"=16711680, "Bold"=TRUE, "Italic"=TRUE, "Underline"=FALSE, "Strikethrough"=FALSE, "Font Encoding"=enum."Cp1252, WinANSI"}  # Bemerkung Font HeaderTable
      w197 = T26 {"Bemerkung Text"="", "Align (Left)"=0, "Add Line Feeds (F:No)"=FALSE, "Font"={"Font"="Arial", "Size"=10, "Colour"=0, "Bold"=FALSE, "Italic"=FALSE, "Underline"=FALSE, "Strikethrough"=FALSE, "Font Encoding"=enum."Cp1252, WinANSI"}} ("Bemerkung")
      w163 = T29 {"Results"=[], "ResultPictures"={"Yes Ctl Refnum"=refnum, "No Ctl Refnum"=refnum}, "use Pictures"=FALSE, "Image Scale (%)"=100.0, "Autoscale? (T)"=TRUE, "Horizontal Align"=3, "Position"=0} ("Results")
      w278 = T27 0 items=["Center", "Justified", "Justified All", "Left", "Right"] ("Align (Left)")
      w247 = T24 {"Font"="Arial", "Size"=26, "Colour"=0, "Bold"=TRUE, "Italic"=FALSE, "Underline"=TRUE, "Strikethrough"=FALSE, "Font Encoding"=enum."Cp1252, WinANSI"}  # Title Font
      w291 = T27 0 items=["Center", "Justified", "Justified All", "Left", "Right"] ("Align (Left)")
      w297 = T27 0 items=["Center", "Justified", "Justified All", "Left", "Right"] ("Align (Left)")
      w187 = T33 {"GraphCtl Refnum"=refnum, "Wrap Text (F:No)"=FALSE, "Hide Grid (F:No)"=FALSE, "Scale (100%)"=0.0, "Align (Left)"=0, "PositionBemerkung"=enum."before", "PageBreak"=enum."after comment"} ("Element")
      w303 = T27 0 items=["Center", "Justified", "Justified All", "Left", "Right"] ("Align (Left)")
      w285 = T5 " - " ("String")
      w194 = T28 {"TableHeader"=["Soll\nppm/%", "Ist\nppm/%", "Fehler\n%", "Toleranz\n%", "Ergebnis"], "Table"=[["aaa", "bbb", "ccc", "ddd"], ["111", "222", "333", "444"], ["sss", "fff", "kkk", "xxx"], ["6.5", "11.13", "19.2", "4"], ["1111", "1212", "777", "888"]], "Relative Column Widths (%)"=[22.5, 22.5, 22.5, 22.5, 4.0], "Results"={"Results"=[], "ResultPictures"={"Yes Ctl Refnum"=refnum, "No Ctl Refnum"=refnum}, "use Pictures"=FALSE, "Image Scale (%)"=100.0, "Autoscale? (T)"=TRUE, "Horizontal Align"=3, "Position"=0}, "PositionBemerkung"=enum."before", "PageBreak"=enum."before", "TablePictures"={"Ctl Refnum In"=[], "RowOrColumn"=enum."Row", "IndexToInsert"=0, "Image Scale (%)"=[], "Autoscale? (T)"=[], "Horizontal Align"=3}, "Horizontal Align"=3} ("Table Array")
      w317 = T27 0 items=["Center", "Justified", "Justified All", "Left", "Right"] ("Align (Left)")
      w318 = 2 ("y")
      # "#PDF_Interface"
      n69 = property on="LIN Ausgabetabelle" class="Tbl (strikt)"() -> (error out=w239:errorcluster, "Column Headers[]"=w204:string[])  [unwired: 2 in, 1 out]
      n70 = for {
        tunnel: w337 -> [w480] mode=indexing
        tunnel: [w481] -> w166 mode=indexing
        tunnel: [w479] -> w165 mode=indexing
        n71 = Select(t="X", s=w480, f="-") -> (s? t:f=w481:string)
        n72 = Bundle("f"=w481, w480) -> (w479:cluster{"f":string, bool})  [unwired: 1 in]
      }
      n73 = Index Array(array=w229, index #1=2 ("Index"), index #2=6 ("Index")) -> (element #1=w332:T5, element #2=w305:T5, element #3=w304:T5)  [unwired: 1 in]
      n74 = Concatenate Strings(w266, T5 ": " ("String")) -> (w281:string)
      n75 = disable-structure shown="Aktiviert" {
        disable-tunnel: w229 -> [w399 w407]
        disable-tunnel: [w398 w406] -> w227
        disable-tunnel: w228 -> [w397 w403]
        disable-tunnel: w226 -> [_ w401]
        frame Disabled {
          n76 = Build Array(w397, w399) -> (w398:T5[][])
        }
        frame Enabled {
          # "Standard Header"
          n77 = Delete From Array(array=w403, length=10 ("Länge"), index=0 ("Index")) -> (array with subset deleted=w402:string[])  [unwired: 1 out]
          n78 = Build Array (concatenate)(w401, w402) -> (w400:string[])
          n79 = Build Array(w400, w407) -> (w406:T5[][])
        }
      }
      n80 = call "FGV_HovaCAL_Interface_AutoLin_MFC.vi"("Aktion"=Aktion_FGV_HovaCAL_Interface_Autolin."lesen") -> ("fix conf"=w213:bool)  [unwired: 7 in, 3 out]
      n81 = call "FGV Gasteiler.vi"("Aktionen"=Aktionen_FGV_Gasteiler_Daten."lesen") -> ("Gasteiler Daten"=w219:T38)  [unwired: 11 in, 7 out]
      n82 = call "SPAN Table.vi"("Sprachliste"=w232, "SpanComponentInfos-Cluster"=w265) -> ("SpanTable Info Array"=w264:string[][])  [unwired: 8 in, 1 out]
      n83 = call "GD and kalibration Infos.vi"("Sprachliste"=w232) -> ("Error occured"=w231:bool, "ErrorMessage PDF"=w230:string)  [unwired: 6 in, 3 out]
      n84 = Unbundle By Name(w219) -> ("Gasteiler Type"=w218:T40)
      n85 = Delete From Array(array=w264, length=1 ("Länge"), index (row)=0 ("Index (Zeile)")) -> (deleted portion=w260:string[][], array with subset deleted=w261:string[][])  [unwired: 1 in]
      n86 = call "Texte in VIs uebersetzen.vi"("Sprachliste"=w206, "String-Array zum Übersetzen"=w204) -> ("String-Array zum Übersetzen"=w202:string[])  [unwired: 9 in, 4 out]
      n87 = Concatenate Strings(w281, w305, w285, w304) -> (w284:string)
      n88 = Bundle By Name(cluster=T35 {"Header Footer Text Cluster"={"Header Text"="Protokoll XYZ", "Footer Text"="IAG nG", "Time"="<TIMESTAMP yyyy-MM-dd>", "Page Number"="Page <P> of <PT>"}, "PDF Details"={"Title"="Test PDF", "Subject"="Versa Tabasco", "Keywords"="", "Author"="RIW", "Creator"="IAG"}} ("Info"), "Header Footer Text Cluster.Header Text"=w251, "PDF Details.Title"=w251, "PDF Details.Author"=w332, "PDF Details.Creator"="IAG nG") -> (w246:T35)
      n89 = Index Array(array=w260) -> (element=w259:string[])  [unwired: 2 in]
      n90 = call "Einheiten in Tabellenspalten Strings.vi"("Fehler (Eingang, kein Fehler)"=w239, "Spalten Titel mit Einheiten in"=w202, "Einheit in"=w237) -> ("Fehler (Ausgang)"=w238:errorcluster, "Spalten Titel mit Einheiten out"=w203:string[])  [unwired: 6 in, 1 out]
      n91 = Equal?(x=w218, y=w217) -> (x = y?=w214:bool)
      n92 = call <vilib>:"Clear Errors.vi"("error in (no error)"=w238) -> ()  [unwired: 5 in, 2 out]
      n93 = Index Array(array=w249) -> (element #1=w196:string, element #2=w195:string, element #3=w191:string, element #4=w184:string, element #5=w182:string)  [unwired: 5 in]
      n94 = Concatenate Strings(w248, w285, w284) -> (w286:string)
      n95 = And(x=w213, y=w214) -> (x .and. y?=w212:bool)
      n96 = Bundle By Name(cluster=T28 {"TableHeader"=[], "Table"=[], "Relative Column Widths (%)"=[], "Results"={"Results"=[], "ResultPictures"={"Yes Ctl Refnum"=refnum, "No Ctl Refnum"=refnum}, "use Pictures"=FALSE, "Image Scale (%)"=0.0, "Autoscale? (T)"=FALSE, "Horizontal Align"=0, "Position"=0}, "PositionBemerkung"=enum."before", "PageBreak"=enum."none", "TablePictures"={"Ctl Refnum In"=[], "RowOrColumn"=enum."Row", "IndexToInsert"=0, "Image Scale (%)"=[], "Autoscale? (T)"=[], "Horizontal Align"=0}, "Horizontal Align"=0} ("Table Array"), "TableHeader"=w259, "Table"=w261, "Relative Column Widths (%)"=sgl[] [10.0, 25.0, 65.0]) -> (w257:T28)
      n97 = Build Array (concatenate)("", w203) -> (w211:string[])
      n98 = Build Array(w191, w184, w182) -> (w183:string[])
      n99 = Bundle By Name(cluster=w163, "Results"=w165, "ResultPictures"=w164, "use Pictures"=TRUE, "Image Scale (%)"=sgl 33.0, "Autoscale? (T)"=FALSE, "Horizontal Align"=w168, "Position"=w161) -> (w167:T29)
      n100 = Bundle By Name(cluster=w197, "Bemerkung Text"=w230, "Align (Left)"=w278, "Add Line Feeds (F:No)"=FALSE, "Font"=w240) -> (w279:T26)
      n101 = Bundle By Name(cluster=w197, "Bemerkung Text"=w284, "Align (Left)"=w303, "Add Line Feeds (F:No)"=FALSE, "Font"=w199) -> (w244:T26)
      n102 = Bundle By Name(cluster=w197, "Bemerkung Text"=w195, "Align (Left)"=w317, "Add Line Feeds (F:No)"=FALSE, "Font"=w199) -> (w280:T26)
      n103 = Bundle By Name(cluster=w197, "Bemerkung Text"=w286, "Align (Left)"=w291, "Add Line Feeds (F:No)"=FALSE, "Font"=w199) -> (w186:T26)
      n104 = Bundle By Name(cluster=w197, "Bemerkung Text"=w196, "Align (Left)"=w201, "Add Line Feeds (F:No)"=FALSE, "Font"=w199) -> (w198:T26)
      n105 = call "Split Deckblatt Table.vi"("Deckblatt"=w224, "Array (Eingang)"=w227, "Numbre of Rows for TitlePage"=6 ("Index (Zeile)")) -> ("HeaderTable"=w270:T5[][], "TitlePage_HeaderTable"=w269:T5[][])  [unwired: 7 in]
      n106 = Transpose 2D Array(2D array=w269) -> (transposed array=w272:T5[][])
      n107 = Subtract(x=100, y=w318) -> (x-y=w321:i32)
      n108 = Build Array(w257) -> (w256:T28[])
      n109 = disable-structure shown="Aktiviert" {
        disable-tunnel: w272 -> [w409 w410]
        disable-tunnel: [w408 w410] -> w271
        frame Disabled {
          n110 = call "Split HeaderTable.vi"("Array (Eingang)"=w409) -> ("Array (Ausgang)"=w408:T5[][])  [unwired: 10 in]
        }
        frame Enabled {
          # "Standard Header"
        }
      }
      n111 = disable-structure shown="Aktiviert" {
        disable-tunnel: w335 -> [w342 w344]
        disable-tunnel: w166 -> [w340 _]
        disable-tunnel: [w339 w344] -> w313
        disable-tunnel: [w338 w343] -> w162
        disable-tunnel: w163 -> [w338 _]
        disable-tunnel: w167 -> [_ w343]
        frame Disabled {
          n112 = Insert Into Array(array=w342, index (col)=0 ("Deaktivierter Index (Spalte)"), new element=w340) -> (w339:string[][])  [unwired: 1 in]
        }
        frame Enabled {
          # "#LIN_Hakerl"
        }
      }
      n113 = Array Size(array=w211) -> (size(s)=w325:i32)
      n114 = call "FGV Referenzen.vi"("Aktikon"=enum16{"lesen", "schreiben"}."lesen") -> ("Referenzen Cluster out"=w154:T60)  [unwired: 8 in, 1 out]
      n115 = Initialize Array(T26 {"Bemerkung Text"="", "Align (Left)"=0, "Add Line Feeds (F:No)"=FALSE, "Font"={"Font"="Arial", "Size"=10, "Colour"=0, "Bold"=FALSE, "Italic"=FALSE, "Underline"=FALSE, "Strikethrough"=FALSE, "Font Encoding"=enum."Cp1252, WinANSI"}} ("Bemerkung"), 2 ("Dimensionsgröße")) -> (w243:T26[])
      n116 = Decrement(x=w325) -> (x-1=w324:i32)
      n117 = Select(t=w279, s=w231, f=w197) -> (s? t:f=w245:T26)
      n118 = Unbundle By Name(w154) -> ("Graphik (Eingang)"=w153:refnum<vi>)
      n119 = Divide(x=w321, y=w324) -> (x/y=w320:dbl)
      n120 = Build Array(w271) -> (w267:T5[][][])
      n121 = Transpose 2D Array(2D array=w270) -> (transposed array=w290:T5[][])
      n122 = for {
        N: w324 -> [_]
        shift-right: [w477] -> w319
        shift-left: sgl[] [] ("Relative Column Widths (%)") -> [w478]
        tunnel: w320 -> [w476]
        n123 = Build Array (concatenate)(w478, w476) -> (w477:dbl[])
      }
      n124 = Build Array(w244, w245, w280, w197, w198, w186, w244) -> (w208:T26[])
      n125 = case shown="True" w212 {
        tunnel: w203 -> [_ w345]
        tunnel: [_ w352] -> w210
        tunnel: w208 -> [_ w351]
        tunnel: [_ w350] -> w207
        tunnel: w205 -> [_ w349]
        frame False {
        }
        frame True {
          # "HovaKAL Komponenten fix"
          n126 = call "PDF HovaCAL fix Tables.vi"("Sprachliste"=w349) -> ("Bemerkungen"=w348:string[], "Eingabetabelle behandelt"=w347:string[][][])  [unwired: 9 in]
          n127 = for {
            tunnel: w345 -> [w364]
            tunnel: [w374] -> w352 mode=indexing
            tunnel: w351 -> [w367]
            tunnel: w348 -> [w365] mode=indexing
            tunnel: w347 -> [w358] mode=indexing
            shift-right: [w363] -> w350
            shift-left: T26[] [] -> [w362]
            n128 = Array Size(array=w364) -> (size(s)=w373:i32)
            n129 = Decrement(x=w373) -> (x-1=w372:i32)
            n130 = Delete From Array(array=w358, length=1 ("Länge"), index (col)=3 ("Index")) -> (array with subset deleted=w355:string[][])  [unwired: 1 in, 1 out]
            n131 = Divide(x=100, y=w372) -> (x/y=w370:dbl)
            n132 = for {
              N: w372 -> [_]
              shift-right: [w379] -> w368
              shift-left: sgl[] [] ("Relative Column Widths (%)") -> [w380]
              tunnel: w370 -> [w378]
              n133 = Build Array (concatenate)(w380, w378) -> (w379:dbl[])
            }
            n134 = Array Subset(array=w355, index (col)=0 ("Index"), length (col)=8 ("Länge")) -> (w354:string[][])  [unwired: 2 in]
            n135 = Bundle By Name(cluster=T28 {"TableHeader"=["Soll\nppm/%", "Ist\nppm/%", "Fehler\n%", "Toleranz\n%", "Ergebnis"], "Table"=[["aaa", "bbb", "ccc", "ddd"], ["111", "222", "333", "444"], ["sss", "fff", "kkk", "xxx"], ["6.5", "11.13", "19.2", "4"], ["1111", "1212", "777", "888"]], "Relative Column Widths (%)"=[22.5, 22.5, 22.5, 22.5, 4.0], "Results"={"Results"=[], "ResultPictures"={"Yes Ctl Refnum"=refnum, "No Ctl Refnum"=refnum}, "use Pictures"=FALSE, "Image Scale (%)"=100.0, "Autoscale? (T)"=TRUE, "Horizontal Align"=3, "Position"=0}, "PositionBemerkung"=enum."before", "PageBreak"=enum."before", "TablePictures"={"Ctl Refnum In"=[], "RowOrColumn"=enum."Row", "IndexToInsert"=0, "Image Scale (%)"=[], "Autoscale? (T)"=[], "Horizontal Align"=3}, "Horizontal Align"=3} ("Table Array"), "TableHeader"=w364, "Table"=w354, "Relative Column Widths (%)"=w368, "PositionBemerkung"=PDFCommentPosition."before", "PageBreak"=PDFPageBreak."none") -> (w374:T28)
            n136 = Index Array(array=w367) -> (element=w366:T26)  [unwired: 1 in]
            n137 = Bundle By Name(cluster=w366, "Bemerkung Text"=w365) -> (w360:T26)
            n138 = Build Array (concatenate)(w362, T26 {"Bemerkung Text"="", "Align (Left)"=0, "Add Line Feeds (F:No)"=FALSE, "Font"={"Font"="Arial", "Size"=10, "Colour"=0, "Bold"=FALSE, "Italic"=FALSE, "Underline"=FALSE, "Strikethrough"=FALSE, "Font Encoding"=enum."Cp1252, WinANSI"}} ("Bemerkung"), w360) -> (w363:T26[])
          }
        }
      }
      n139 = And(x=w174, y=w172) -> (x .and. y?=w173:bool)
      n140 = Bundle By Name(cluster=T31 {"Titel"="Test mit Graph PDF", "Header Tables"=[[["Murks:", "4711"], ["HolyShit:", "0815"]]], "Bemerkungen"=[]} ("Content"), "Titel"=w251, "Header Tables"=w267, "Bemerkungen"=w243) -> (w273:T31)
      n141 = Or(x=w235, y=w173) -> (x .or. y?=w175:bool)
      n142 = Build Array(w178, w181, w180) -> (w179:T5[][])
      n143 = Transpose 2D Array(2D array=w179) -> (transposed array=w177:T5[][])
      n144 = Build Array(w160) -> (w310:string[][])
      n145 = Bundle By Name(cluster=w158, "Scale (100%)"=sgl 55.0, "GraphCtl Refnum"=w153) -> (w159:T33)
      n146 = disable-structure shown="Aktiviert" {
        disable-tunnel: [w395 w396] -> w225
        disable-tunnel: w176 -> [_ w396]
        frame Disabled {
          w395 = sgl[] [35.0, 35.0]  # Column Ratio left
        }
        frame Enabled {
          (unwired) sgl[] [50.0, 50.0]  # Column Ratio left
          # "Standard Header"
        }
      }
      n147 = Initialize Array(sgl 20.0, 5 ("Dimensionsgröße")) -> (w307:sgl[])
      n148 = Build Array (concatenate)(w318, w319) -> (w315:dbl[])
      n149 = case shown="True" w224 {
        tunnel: w290 -> [w391 w394]
        tunnel: [w391 w393] -> w289
        tunnel: [w390 w392] -> w223
        tunnel: w176 -> [w390 _]
        frame False {
          (unwired) sgl[] [40.0, 60.0]  # Column Ratio left
        }
        frame True {
          w392 = sgl[] [40.0, 60.0, 80.0, 20.0]  # Column Ratio left
          n150 = call "Split HeaderTable.vi"("Array (Eingang)"=w394) -> ("Array (Ausgang)"=w393:T5[][])  [unwired: 10 in]
        }
      }
      n151 = Bundle By Name(cluster=w194, "TableHeader"=w211, "Table"=w313, "Relative Column Widths (%)"=w315, "Results"=w162, "PositionBemerkung"=PDFCommentPosition."before", "PageBreak"=PDFPageBreak."before") -> (w312:T28)
      n152 = Bundle By Name(cluster=w194, "TableHeader"=w183, "Table"=w177, "Relative Column Widths (%)"=sgl[] [76.0, 12.0, 12.0], "Results"=w163, "PositionBemerkung"=PDFCommentPosition."before", "PageBreak"=PDFPageBreak."none") -> (w190:T28)
      n153 = Bundle By Name(cluster=w194, "TableHeader"=w250, "Table"=w310, "Relative Column Widths (%)"=w307, "Results"=w163, "PositionBemerkung"=PDFCommentPosition."before", "PageBreak"=PDFPageBreak."none") -> (w311:T28)
      n154 = Select(t=w159, s=w156, f=w158) -> (s? t:f=w157:T33)
      n155 = Build Array(T24 {"Font"="Arial", "Size"=10, "Colour"=0, "Bold"=FALSE, "Italic"=FALSE, "Underline"=FALSE, "Strikethrough"=FALSE, "Font Encoding"=enum."Cp1252, WinANSI"} ("HeaderTableFont")) -> (w254:T24[])
      n156 = case shown="True" w175 {
        tunnel: w246 -> [_ w421]
        tunnel: w288 -> [w413 w430]
        tunnel: [w412 w437] -> w276
        tunnel: [w411 w436] -> w275
        tunnel: w224 -> [_ w419]
        tunnel: w247 -> [_ w435]
        tunnel: w273 -> [_ w434]
        tunnel: w256 -> [_ w432]
        tunnel: w254 -> [_ w431]
        tunnel: w174 -> [_ w428]
        tunnel: w236 -> [_ w425]
        tunnel: w235 -> [_ w424]
        tunnel: w234 -> [_ w423]
        tunnel: w233 -> [_ w422]
        tunnel: w225 -> [_ w420]
        tunnel: w172 -> [_ w416]
        tunnel: w157 -> [_ w415]
        frame False {
          n157 = call <vilib>:"SAI_PDF_New Page.vi"("error in"=w413, "Context In"="Context (Eingang)") -> ("error out"=w411:errorcluster, "Context Out"=w412:refnum<class "Context.lvclass">)  [unwired: 8 in]
        }
        frame True {
          n158 = Compound Arithmetic op=AND ("Mehrfacharithmetik")(w428, w424, w419, w416) -> (w418:bool)
          n159 = call "Logos.vi"("Fehler (Eingang, kein Fehler)"=w430) -> ("Fehler (Ausgang)"=w429:errorcluster, "Footer Image File Path"=w440:path, "Header Image File Path"=w441:path)  [unwired: 7 in, 1 out]
          n160 = call "Deckblatt_Filename.vi"("Deckblatt Filename"=w422, "Deckblatt Prefix"=w423, "PDF Einzelseiten & Start"=w418, "Save PDF File Path (Eingang)"="Save PDF File Path") -> ("PDF Einzelseiten & Start out"=w417:bool, "Save PDF File Path (Ausgang)"=w427:path)  [unwired: 6 in]
          n161 = call "InitBeforePage.vi"("Info"=w421, "Fehler (Eingang, kein Fehler)"=w429, "Footer Image File Path"=w440, "Header Image File Path"=w441, "Path (Dialog if Empty)"=w427) -> ("Fehler (Ausgang)"=w438:errorcluster, "Context (Ausgang)"=w439:refnum<class "Context.lvclass">)  [unwired: 5 in]
          n162 = Build Array(w420) -> (w433:sgl[][])
          n163 = case shown="True" w419 {
            tunnel: w439 -> [w443 w448]
            tunnel: [w443 w450] -> w437
            tunnel: w438 -> [w442 w459]
            tunnel: [w442 w451] -> w436
            tunnel: w435 -> [_ w458]
            tunnel: w434 -> [_ w457]
            tunnel: w433 -> [_ w456]
            tunnel: w432 -> [_ w455]
            tunnel: w431 -> [_ w454]
            tunnel: w417 -> [_ w449]
            tunnel: "Save PDF File Path" -> [_ w447]
            tunnel: w425 -> [_ w446]
            tunnel: w421 -> [_ w445]
            tunnel: w415 -> [_ w444]
            frame False {
            }
            frame True {
              n164 = call "TitlePage.vi"("Graph"=w444, "HeaderTableFonts"=w454, "Title Font"=w458, "Column Ratios left"=w456, "error in"=w459, "Table Array"=w455, "Content"=w457, "Context (Eingang)"=w448) -> ("error out"=w452:errorcluster, "Context (Ausgang)"=w453:refnum<class "Context.lvclass">)  [unwired: 2 in]
              n165 = case shown="True" w449 {
                tunnel: w453 -> [w461 w472]
                tunnel: w452 -> [w460 w471]
                tunnel: [w460 w469] -> w451
                tunnel: [w461 w470] -> w450
                tunnel: w447 -> [_ w468]
                tunnel: w446 -> [_ w463]
                tunnel: w445 -> [_ w462]
                frame False {
                }
                frame True {
                  n166 = call "ClosePage.vi"("popup viewer"=w463, "Fehler (Eingang, kein Fehler)"=w471, "Context (Eingang)"=w472) -> ("Fehler (Ausgang)"=w465:errorcluster)  [unwired: 8 in]
                  n167 = call "Logos.vi"("Fehler (Eingang, kein Fehler)"=w465) -> ("Fehler (Ausgang)"=w464:errorcluster, "Footer Image File Path"=w466:path, "Header Image File Path"=w467:path)  [unwired: 7 in, 1 out]
                  n168 = call "InitBeforePage.vi"("Info"=w462, "Fehler (Eingang, kein Fehler)"=w464, "Footer Image File Path"=w466, "Header Image File Path"=w467, "Path (Dialog if Empty)"=w468) -> ("Fehler (Ausgang)"=w469:errorcluster, "Context (Ausgang)"=w470:refnum<class "Context.lvclass">)  [unwired: 5 in]
                }
              }
            }
          }
        }
      }
      n169 = disable-structure shown="Aktiviert" {
        disable-tunnel: [w473 "XY-Graph LIN" w475] -> w329
        frame Disabled {
          n170 = control-ref of="XY-Graph LIN"() -> (w473:refnum<vi>)
        }
        frame Enabled {
        }
        frame Disabled {
        }
      }
      n171 = Build Array(w189, T24 {"Font"="Arial", "Size"=8, "Colour"=0, "Bold"=FALSE, "Italic"=FALSE, "Underline"=FALSE, "Strikethrough"=FALSE, "Font Encoding"=enum."Cp1252, WinANSI"} ("TableFont"), w189) -> (w221:T24[])
      n172 = case shown="True" w212 {
        tunnel: w312 -> [w383 w389]
        tunnel: [w381 w388] -> w220
        tunnel: w210 -> [_ w387]
        tunnel: w208 -> [w382 w386]
        tunnel: [w382 w385] -> w209
        tunnel: w207 -> [_ w384]
        frame False {
          n173 = Build Array(w383) -> (w381:T28[])
        }
        frame True {
          n174 = Build Array (concatenate)(w389, w387) -> (w388:T28[])
          n175 = Build Array (concatenate)(w386, w384) -> (w385:T26[])
        }
      }
      n176 = Build Array (concatenate)(w190, w311, w220) -> (w314:T28[])
      n177 = Bundle By Name(cluster=T33 {"GraphCtl Refnum"=refnum, "Wrap Text (F:No)"=FALSE, "Hide Grid (F:No)"=FALSE, "Scale (100%)"=100.0, "Align (Left)"=0, "PositionBemerkung"=enum."before", "PageBreak"=enum."after comment"} ("Graph"), "GraphCtl Refnum"=w329, "Scale (100%)"=sgl 33.0, "Align (Left)"=w297, "PositionBemerkung"=PDFCommentPosition."after", "PageBreak"=PDFPageBreak."none", "Hide Grid (F:No)"=TRUE) -> (w188:T33)
      n178 = Bundle By Name(cluster=T32 {"Titel"="", "Header Table"=[], "Table Array"=[], "Bemerkungen"=[]} ("Content"), "Titel"=w251, "Header Table"=w289, "Table Array"=w314, "Bemerkungen"=w209) -> (w326:T32)
      n179 = Build Array(w187, w188, w187) -> (w316:T33[])
      n180 = call "AddPageContent.vi"("Graph last"=TRUE, "Deckblatt"=w224, "TableFont"=w221, "Title Font"=w247, "Column Ratio left"=w223, "error in"=w275, "Graph Array"=w316, "Content"=w326, "Context (Eingang)"=w276) -> ("error out"=w328:errorcluster, "Context (Ausgang)"=w287:refnum<class "Context.lvclass">)  [unwired: 1 in]
    }
    frame #3 {
      # "#PDF_Interface"
      n181 = disable-structure shown="Deaktiviert" {
        frame Disabled {
          n182 = vi-ref "PDF_Interface_PDF Protokoll Linearisierung.vi"() -> (w484:refnum<vi>)
          n183 = call "VI Shut Down.vi"("VI Referenz"=w484) -> ()  [unwired: 11 in]
        }
        frame Enabled {
        }
      }
    }
  }
  "error out" <- w34
  "Context (Ausgang)" <- w33
